vi "Read Manifold Parameters (Purdue).vi"(8 "error in":errorcluster, 11 "Config Manager in":refnum<class "Config Manager Class.lvclass">) -> (0 "error out":errorcluster, 2 "Channel":i32, 3 "Config Manager out":refnum<class "Config Manager Class.lvclass">)   [LabVIEW 2011, in "Config Manager Class.lvclass"]
uses:
  Config Manager Class.lvclass
  <vilib>/Utility/config.llb/NI_LVConfig.lvlib
  <vilib>/Utility/config.llb/Read Key (I32).vi
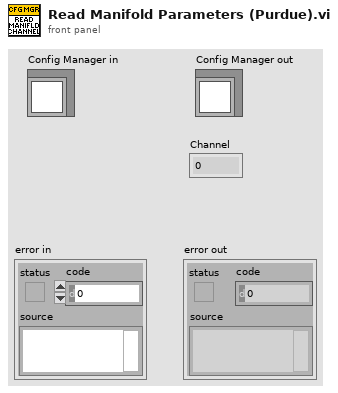
[diagram p1: front panel]
types:
  T1 = typedef "NI_LVConfig.lvlib/Config Data RefNum.ctl" = refnum<k1>
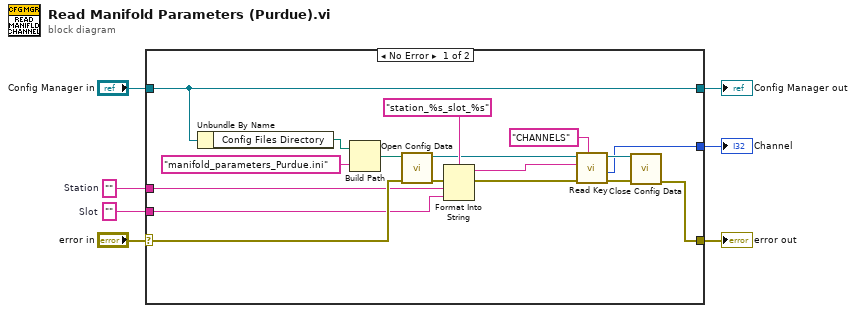
[diagram p0: block diagram]
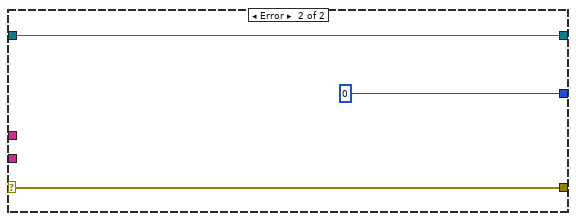
[diagram p2: hidden frame]
diagram:
  w1 = ""  # Slot
  w2 = ""  # Station
  n1 = case shown="No Error" "error in" {
    selector: "error in" -> [w16 w27]
    tunnel: [w11 w27] -> w6
    tunnel: [w19 w26] -> w4
    tunnel: "Config Manager in" -> [w19 w26]
    tunnel: [w10 0 ("value")] -> w3
    tunnel: w2 -> [w9 _]
    tunnel: w1 -> [w8 _]
    frame No Error {
      n2 = Unbundle By Name(w19) -> ("Config Files Directory"=w18:path)
      n3 = Build Path(base path=w18, name or relative path="manifold_parameters_Purdue.ini") -> (appended path=w17:path)
      n4 = call <vilib>:"Open Config Data.vi"("error in (no error)"=w16, "configuration file path"=w17) -> ("error out"=w15:errorcluster, "refnum"=w14:T1)  [unwired: 7 in, 1 out]
      n5 = Format Into String(format string="station_%s_slot_%s", error in=w15, w9, w8) -> (resulting string=w21:string, error out=w22:errorcluster)  [unwired: 1 in]
      n6 = call-poly <vilib>:"Read Key.vi"("section"="CHANNELS", "error in (no error)"=w22, "key"=w21, "refnum"=w14) -> ("error out"=w12:errorcluster, "value"=w10:i32, "refnum out"=w13:T1)  [unwired: 4 in, 1 out]
      n7 = call <vilib>:"Close Config Data.vi"("error in (no error)"=w12, "refnum"=w13) -> ("error out"=w11:errorcluster)  [unwired: 8 in, 1 out]
    }
    frame Error {
    }
  }
  "error out" <- w6
  "Config Manager out" <- w4
  "Channel" <- w3
